vi "Configure Current.vi"(0 "VISA resource name":refnum<visa-resource-name>, 1 "Triggered Peak Current Limit (13 A)":dbl=13.0 format="%#.4g", 5 "Current Range (28.5671 A)":dbl=28.5671 format="%#.4g", 7 "Enable RMS Current Limit (F: Disable)":bool, 9 "RMS Current Limit (1 A)":dbl=1.0 format="%#.4g", 11 "error in (no error)":errorcluster, 12 "Peak Current Limit (13 A)":dbl=13.0 format="%#.4g", 13 "Peak Current Limit Mode (0: Fixed)":u16(ring) items=["Fixed", "Step", "Pulse", "List"]) -> (4 "VISA resource name out":refnum<visa-resource-name>, 15 "error out":errorcluster)   [LabVIEW 2020, in "Agilent 681x Series.lvlib"]
doc: "Configures the current settings of the instrument."
uses:
  <instrlib>/Agilent 681x Series/Agilent 681x Series.lvlib
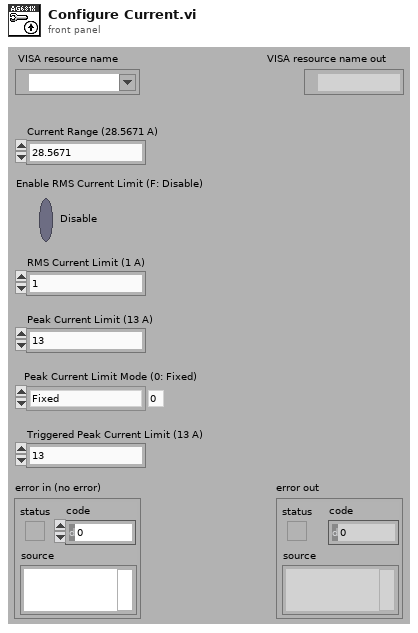
[diagram p1: front panel]
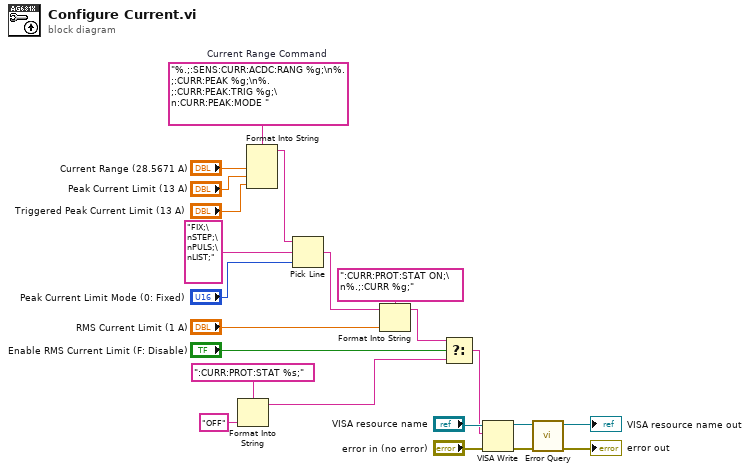
[diagram p0: block diagram]
diagram:
  w18 = "%.;:SENS:CURR:ACDC:RANG %g;\n%.;:CURR:PEAK %g;\n%.;:CURR:PEAK:TRIG %g;\n:CURR:PEAK:MODE "  # Current Range Command
  n1 = Format Into String(format string=":CURR:PROT:STAT %s;", "OFF" ("input 1")) -> (resulting string=w3:string)  [unwired: 2 in, 1 out]
  n2 = Format Into String(format string=w18, "Current Range (28.5671 A)", "Peak Current Limit (13 A)", "Triggered Peak Current Limit (13 A)") -> (resulting string=w14:string)  [unwired: 2 in, 1 out]
  n3 = Pick Line(string ("")=w14, multi-line string="FIX;\nSTEP;\nPULS;\nLIST;", line index="Peak Current Limit Mode (0: Fixed)") -> (output string=w8:string)
  n4 = Format Into String(format string=":CURR:PROT:STAT ON;\n%.;:CURR %g;", initial string=w8, "RMS Current Limit (1 A)") -> (resulting string=w2:string)  [unwired: 1 in, 1 out]
  n5 = Select(t=w2, s="Enable RMS Current Limit (F: Disable)", f=w3) -> (s? t:f=w9:string)
  n6 = VISA Write(VISA resource name="VISA resource name", write buffer=w9, error in (no error)="error in (no error)") -> (VISA resource name out=w20:refnum<visa-resource-name>, error out=w19:errorcluster)  [unwired: 1 out]
  n7 = call <instrlib>:"Error Query.vi"("error in (no error)"=w19, "VISA resource name"=w20) -> ("error out"=→"error out":errorcluster, "VISA resource name out"=→"VISA resource name out":refnum<visa-resource-name>)  [unwired: 6 in, 2 out]
